vi "Auto.vi"() -> ()   [LabVIEW 2020]
uses:
  Global_Variable/Global.vi
  Global_Variable/A180648.vi
  Global_Variable/System_Conf.vi
  Libraries/S7/S7.lvlib
panel:
  out "前序":string
  out "用户事件输出":refnum<user-event>
  out "磨合正向初始化":bool
  out "工位三开始计时1":bool
  out "产品变更_Event":refnum<user-event>
  out "T1+T2":dbl
  out "T2":dbl
  out "T1":dbl
  out "吸收电流":sgl
  out "输出扭矩(大)":sgl
  out "输入扭矩":sgl
  out "力特性逆向去程":bool
  out "力特性正向去程":bool
  out "力特性逆向回程":bool
  out "力特性正向回程":bool
  out "工位三开始计时":bool
  out "工位二开始计时":bool
  out "功能正向初始化":bool
  out "功能逆向初始化":bool
  out "空载逆向初始化":bool
  out "空载正向初始化":bool
  out "试验项目":T1(tab)
  out "拉压曲线":cluster{dbl[], dbl[]}[](graph)
  out "侧铆曲线":cluster{dbl[], dbl[]}[](graph)
  out "0°曲线":cluster{dbl[], dbl[]}[](graph)
  out "45°曲线":cluster{dbl[], dbl[]}[](graph)
  out "力特性试验":cluster{dbl[], dbl[]}[](graph)
  out "功能试验":cluster{dbl[], dbl[]}[](graph)
  out "电流特性试验":cluster{dbl[], dbl[]}[](graph)
  out "逆向空载试验":cluster{dbl[], dbl[]}[](graph)
  out "磨合":cluster{dbl[], dbl[]}[](graph)
  in  "判定结果":bool[][](array[boolean])=[[TRUE]]
  in  "STEP":string
  # "车速0"
  # "车速1"
  # "车速2"
  # "车速3"
  # "车速4"
  # "车速5"
  # "车速0"
  # "车速1"
  # "车速2"
  # "车速3"
  # "车速4"
  # "车速5"
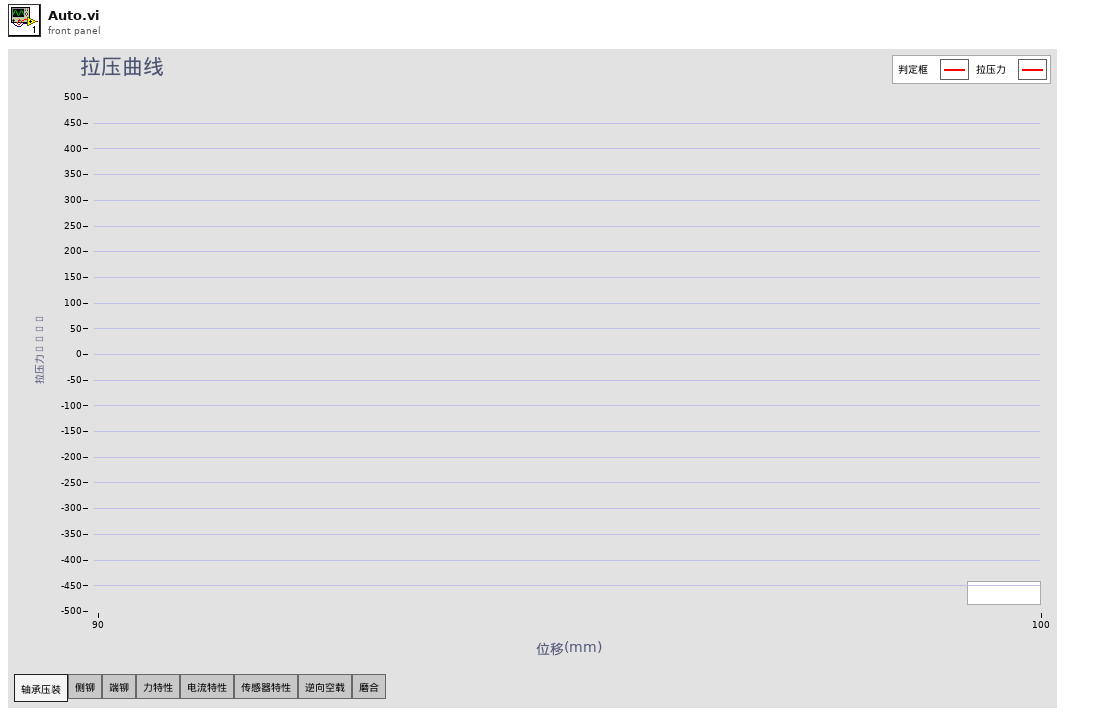
[diagram p1: front panel]
types:
  T1 = enum32{"轴承压装", "侧铆", "端铆", "力特性", "电流特性", "传感器特性", "逆向空载", "磨合"}
  T2 = enum32{"Invalid", "Standard", "Closed", "Hidden", "Minimized", "Maximized"}
  T3 = cluster{"输入轴扭矩":dbl, "输出轴扭矩小量程":dbl, "输出轴扭矩大量程":dbl}
  T4 = typedef "System_conf.ctl" = cluster{"空载滤波":bool, "逆向空载滤波":bool, "空载扭矩系数":dbl, "逆向空载扭矩系数":dbl}
  T5 = cluster{"位移":cluster{"单位":string, "下限":dbl, "上限":dbl}, "压力":cluster{"单位":string, "下限":dbl, "上限":dbl}}
  T6 = cluster{"压最大值":cluster{"单位":string, "下限":dbl, "上限":dbl}, "压力最小值":cluster{"单位":string, "下限":dbl, "上限":dbl}, "拉力最大值":cluster{"单位":string, "下限":dbl, "上限":dbl}, "拉力最小值":cluster{"单位":string, "下限":dbl, "上限":dbl}}
  T7 = cluster{"输入旋转位移":sgl, "电缸位移":sgl, "工装移载位移":sgl, "电缸位移":sgl, "输入扭矩":sgl, "拉压力":sgl, "输出扭矩(大)":sgl, "电缸压力":sgl}
  T8 = typedef "lveventtype.ctl" = enum32{"Null", "Timeout", "Annotation Menu Selection", "Annotation Menu Selection?", "App Instance Close", "App Instance Close?", "Autoscale Range Change", "Bookmark Info Change", "Cell Edit", "Cell Edit?", "Cursor Grab", "Cursor Grab?", "Cursor Menu Selection", "Cursor Menu Selection?", "Cursor Move", "Cursor Release", "Data Change", "Direction Change", "Display State Change", "Drag Ended", "Drag Enter", "Drag Leave", "Drag Over", "Drag Source Update", "Drag Starting", "Drag Starting?", "Drop", "Exec State Change", "Key Down", "Key Down?", "Key Repeat", "Key Repeat?", "Key Up", "Listbox Double Click", "Menu Activation?", "Menu Selection (App)", "Menu Selection? (App)", "Menu Selection (User)", "Mouse Down", "Mouse Down?", "Mouse Enter", "Mouse Leave", "Mouse Move", "Mouse Up", "Mouse Wheel", "NI Security User Change (App)", "Pane Size", "Panel Close", "Panel Close?", "Panel Resize", "Plot Attribute Change", "Scale Range Change", "Shortcut Menu Activation?", "Shortcut Menu Selection (App)", "Shortcut Menu Selection? (App)", "Shortcut Menu Selection (User)", "Tree Double Click", "Tree Drag", "Tree Drag?", "Tree Drop", "Tree Drop?", "Tree Item Close", "Tree Item Close?", "Tree Item Open", "Tree Item Open?", "User Event", "Value Change"}
  T9 = typedef "LVPoint32TypeDef.ctl" = cluster{"Horizontal":i32, "Vertical":i32}
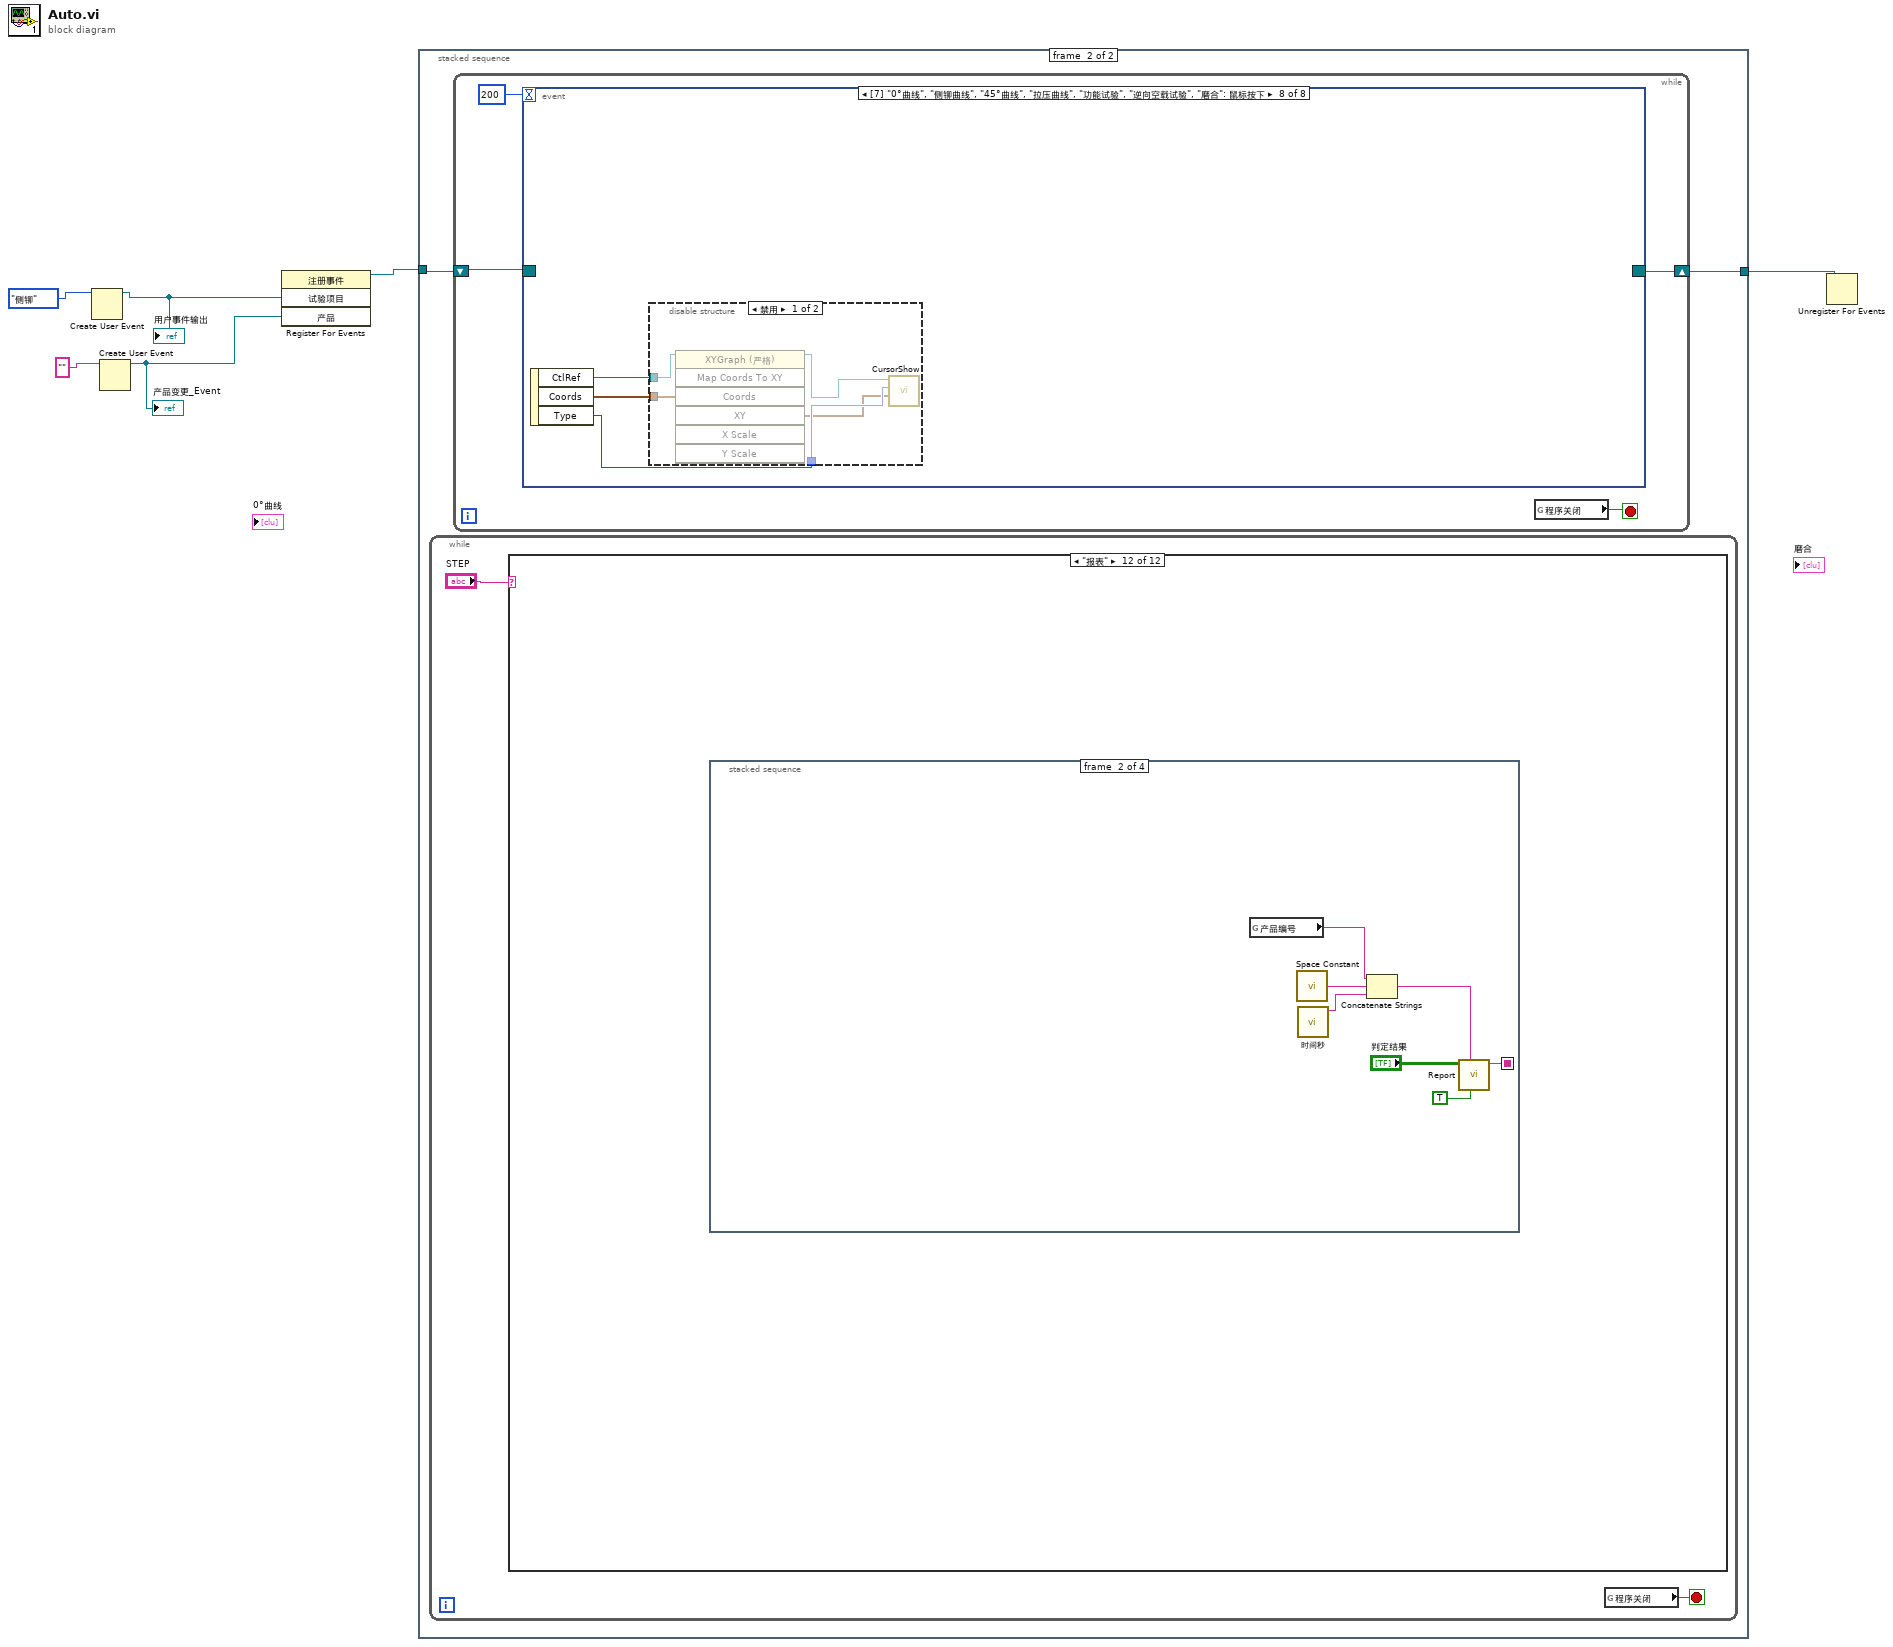
[diagram p0: block diagram]
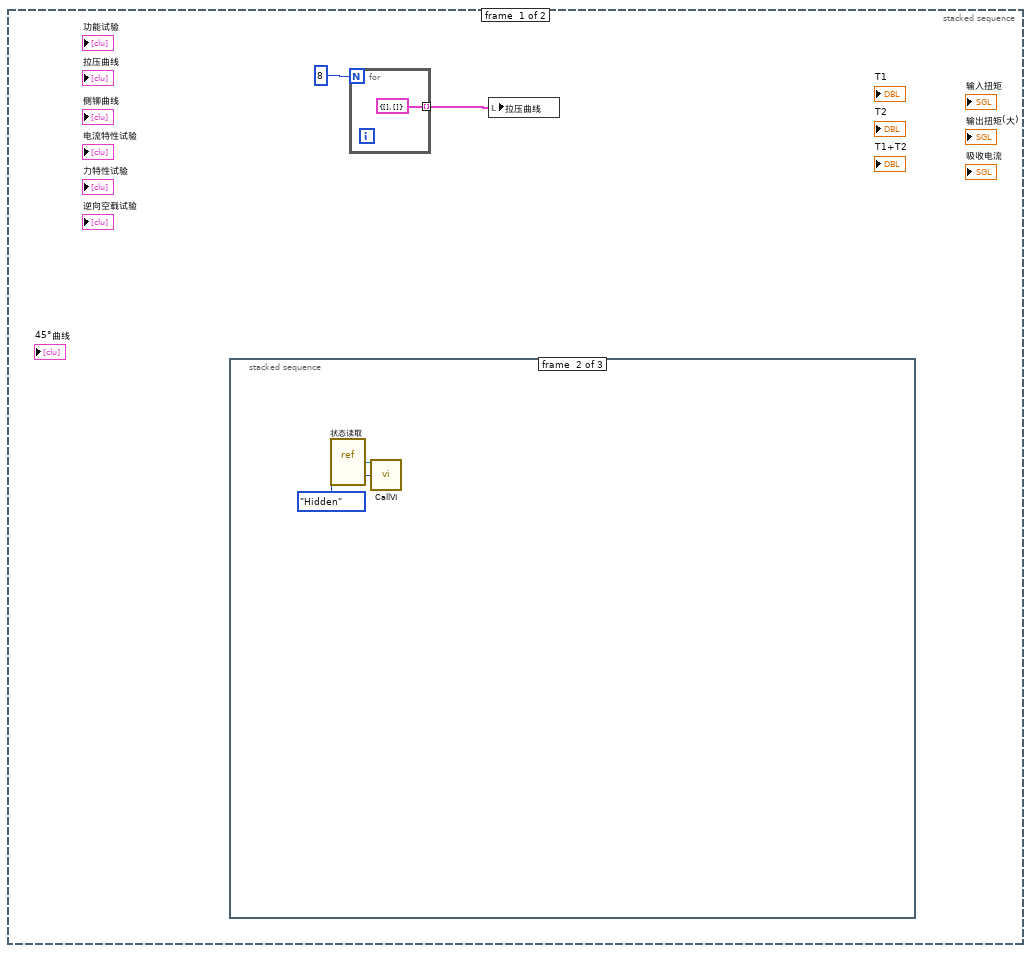
[diagram p2: hidden frame]
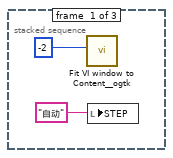
[diagram p3: hidden frame]
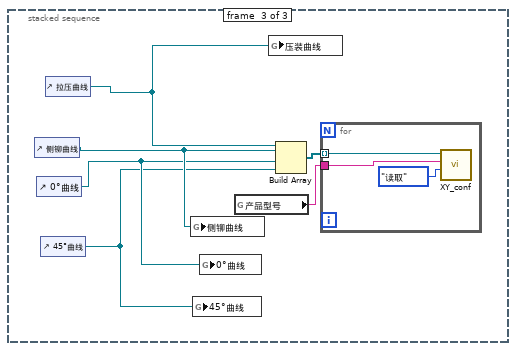
[diagram p4: hidden frame]
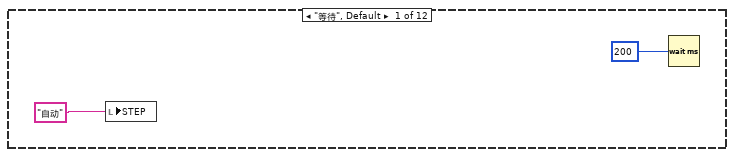
[diagram p5: hidden frame]
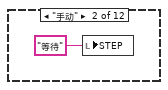
[diagram p6: hidden frame]
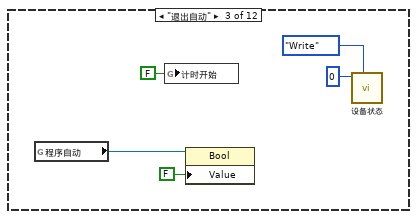
[diagram p7: hidden frame]
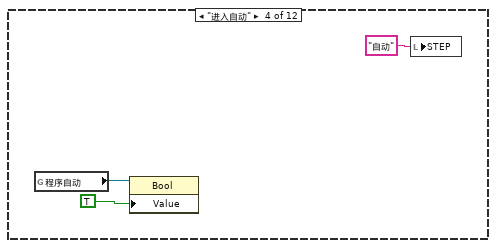
[diagram p8: hidden frame]
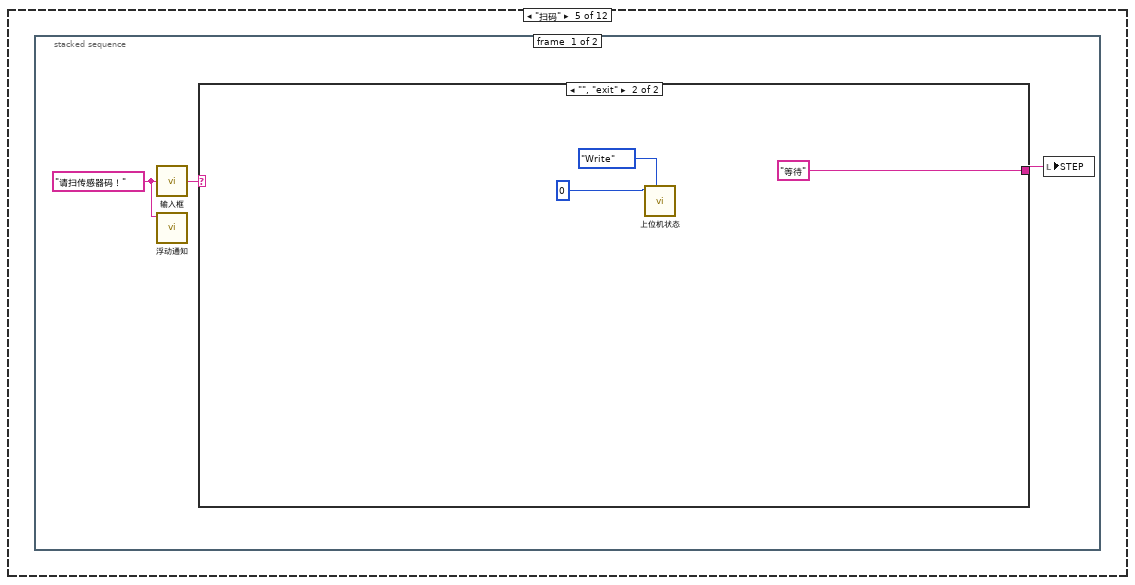
[diagram p9: hidden frame]
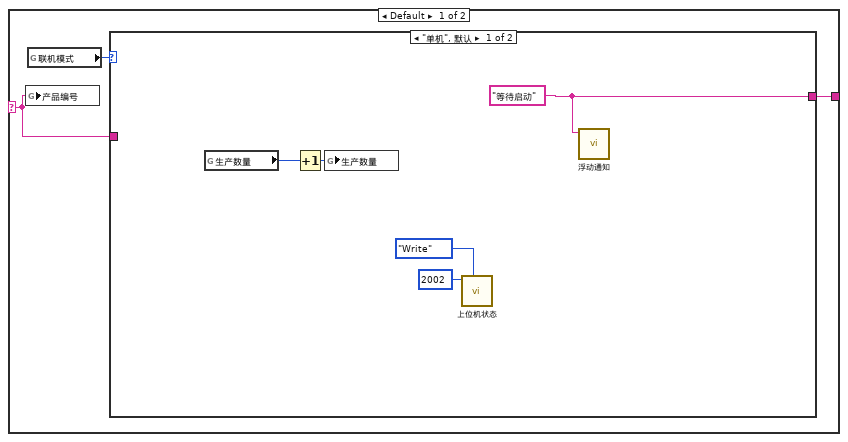
[diagram p10: hidden frame]
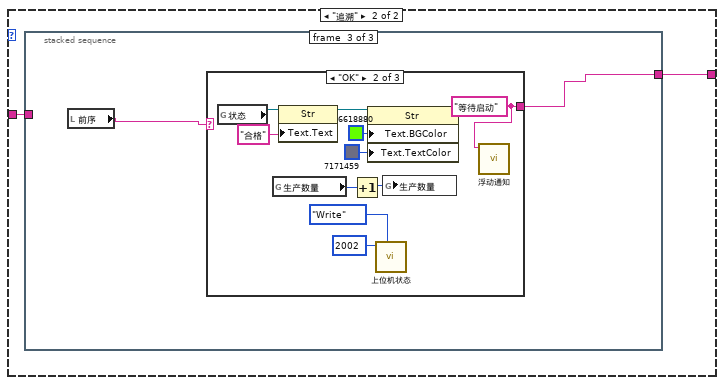
[diagram p11: hidden frame]
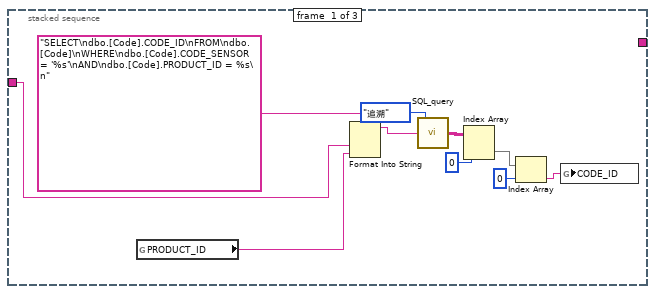
[diagram p12: hidden frame]
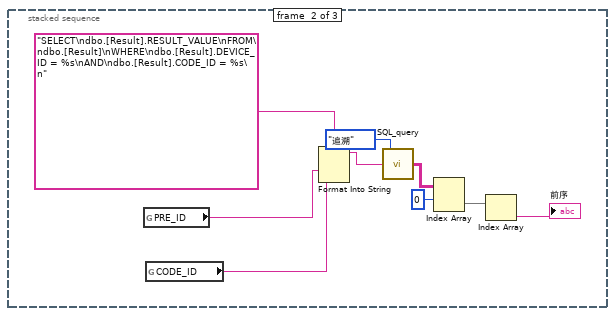
[diagram p13: hidden frame]
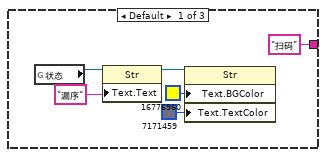
[diagram p14: hidden frame]
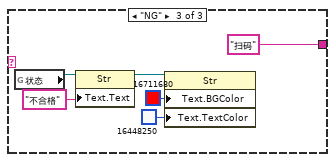
[diagram p15: hidden frame]
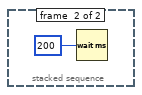
[diagram p16: hidden frame]
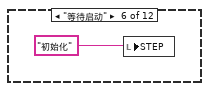
[diagram p17: hidden frame]
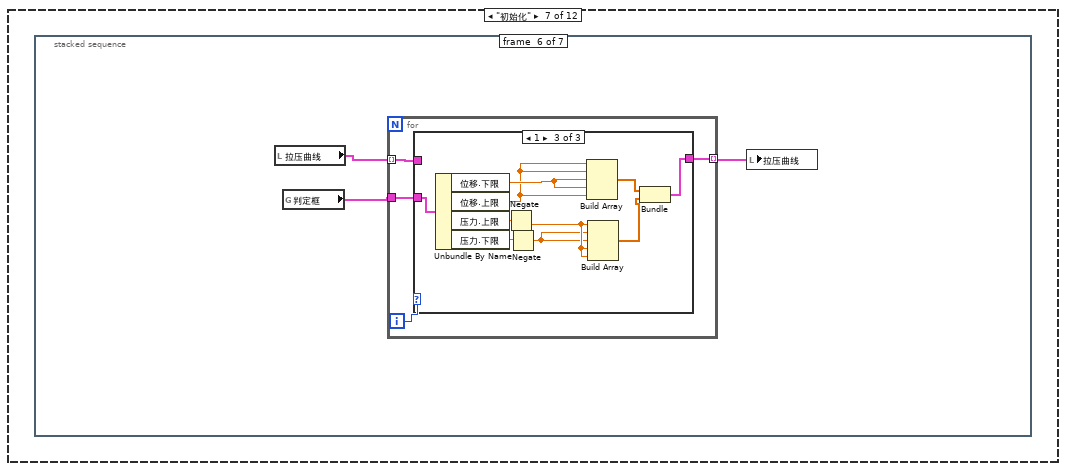
[diagram p18: hidden frame]
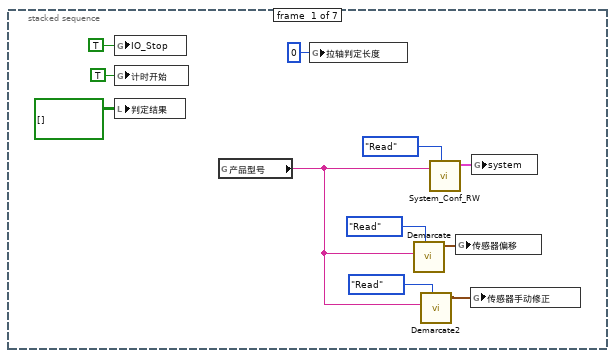
[diagram p19: hidden frame]
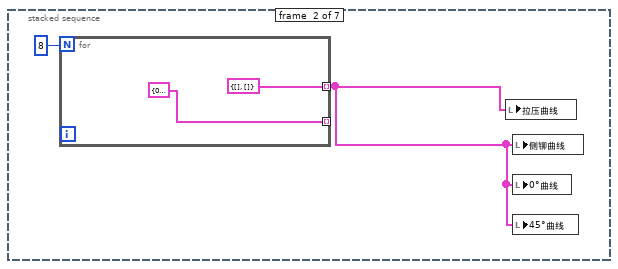
[diagram p20: hidden frame]
diagram:
  n1 = Create User Event(user event datatype=T1."侧铆" ("试验项目")) -> (user event=w1:refnum<user-event>)  [unwired: 1 in, 1 out]
  "用户事件输出" <- w1
  n2 = Create User Event(user event datatype="" ("产品")) -> (user event=w3:refnum<user-event>)  [unwired: 1 in, 1 out]
  "产品变更_Event" <- w3
  n3 = register-events(w1, w3) -> (reference out=w6:refnum<event-registration>)  [unwired: 2 in, 1 out]
  n4 = stacked-sequence {
    tunnel: w6 -> [_ w24]
    tunnel: [_ w23] -> w5
    frame #0 {
      n5 = stacked-sequence {
        frame #0 {
          n6 = call <userlib>:"Fit VI window to Content__ogtk.vi"("border spacing (2 px)"=-2) -> ()  [unwired: 5 in, 2 out]
          n7 = local write "STEP"("自动" ("STEP")) -> ()
        }
        frame #1 {
          n8 = vi-ref "状态读取.vi"() -> (w13:refnum<vi>)
          n9 = call "CallVI.vi"("VI引用"=w13, "状态"=T2."Hidden") -> ()  [unwired: 12 in, 2 out]
        }
        frame #2 {
          n10 = control-ref of="侧铆曲线"() -> (w17:refnum<vi>)
          n11 = control-ref of="0°曲线"() -> (w16:refnum<vi>)
          n12 = control-ref of="45°曲线"() -> (w15:refnum<vi>)
          n13 = control-ref of="拉压曲线"() -> (w14:refnum<vi>)
          n14 = global write "A180648.vi" "侧铆曲线"(w17) -> ()
          n15 = global write "A180648.vi" "45°曲线"(w15) -> ()
          n16 = global write "A180648.vi" "0°曲线"(w16) -> ()
          n17 = global read "Global.vi" "产品型号"() -> (w18:string)
          n18 = global write "A180648.vi" "压装曲线"(w14) -> ()
          n19 = Build Array(w14, w17, w16, w15) -> (w19:refnum<vi>[])
          n20 = for {
            tunnel: w19 -> [w21] mode=indexing
            tunnel: w18 -> [w20]
            n21 = call "XY_conf.vi"("方式"=enum16{"写入", "读取"}."读取", "产品"=w20, "XY图引用"=w21) -> ()  [unwired: 4 in, 1 out]
          }
        }
      }
      n22 = for {
        N: 8 -> [_]
        tunnel: [cluster{dbl[], dbl[]} {[], []}] -> w8 mode=indexing
      }
      n23 = local write "拉压曲线"(w8) -> ()
    }
    frame #1 {
      n24 = while {
        stop <- w26 stop-if-true
        n25 = case shown="\"报表\"" "STEP" {
          frame "等待", Default {
            n26 = local write "STEP"("自动" ("STEP")) -> ()
            n27 = Wait (ms)(milliseconds to wait=u32 200 ("等待时间（毫秒）")) -> ()  [unwired: 1 out]
          }
          frame "手动" {
            n28 = local write "STEP"("等待" ("STEP")) -> ()
          }
          frame "退出自动" {
            n29 = global read "Global.vi" "程序自动"() -> (w31:refnum<vi>)
            n30 = global write "Global.vi" "计时开始"(FALSE ("计时开始")) -> ()
            n31 = property class="Bool"(reference=w31, "Value"=FALSE) -> ()  [unwired: 1 in, 2 out]
            n32 = call "设备状态.vi"("枚举"=enum16{"Read", "Write"}."Write", "Status_Write"=i16 0) -> ()  [unwired: 9 in, 1 out]
          }
          frame "进入自动" {
            n33 = global read "Global.vi" "程序自动"() -> (w36:refnum<vi>)
            n34 = property class="Bool"(reference=w36, "Value"=TRUE) -> ()  [unwired: 1 in, 2 out]
            n35 = local write "STEP"("自动" ("STEP")) -> ()
          }
          frame "扫码" {
            n36 = stacked-sequence {
              frame #0 {
                w39 = "请扫传感器码！" ("提示信息")
                n37 = call "输入框.vi"("提示信息"=w39) -> ("条形码输出"=w40:string)
                n38 = call "浮动通知.vi"("通知内容"=w39) -> ()  [unwired: 11 in]
                n39 = case shown="\"\", \"exit\"" w40 {
                  selector: w40 -> [w41 _]
                  tunnel: [w43 "等待" ("State(s) in Front (\"\")")] -> w38
                  frame Default {
                    n40 = global write "Global.vi" "产品编号"(w41) -> ()
                    n41 = global read "Global.vi" "联机模式"() -> (w42:enum16{"单机", "追溯"})
                    n42 = case shown="\"单机\", 默认" w42 {
                      tunnel: [w46 w50] -> w43
                      tunnel: w41 -> [_ w49]
                      frame "单机", Default {
                        w46 = "等待启动" ("State(s) in Front (\"\")")
                        n43 = global read "Global.vi" "生产数量"() -> (w47:i32)
                        n44 = Increment(x=w47) -> (x+1=w48:i32)
                        n45 = global write "Global.vi" "生产数量"(w48) -> ()
                        n46 = call "上位机状态.vi"("枚举"=enum16{"Read", "Write"}."Write", "Status_Write"=i16 2002) -> ()  [unwired: 9 in, 1 out]
                        n47 = call "浮动通知.vi"("通知内容"=w46) -> ()  [unwired: 11 in]
                      }
                      frame "追溯" {
                        n48 = stacked-sequence {
                          tunnel: [_ _ w71] -> w50
                          tunnel: w49 -> [w59 _ _]
                          frame #0 {
                            n49 = global read "追溯Global.vi" "PRODUCT_ID"() -> (w58:string)
                            n50 = Format Into String(format string="SELECT\ndbo.[Code].CODE_ID\nFROM\ndbo.[Code]\nWHERE\ndbo.[Code].CODE_SENSOR = '%s'\nAND\ndbo.[Code].PRODUCT_ID = %s\n" ("格式字符串"), w59, w58) -> (resulting string=w57:string)  [unwired: 2 in, 1 out]
                            n51 = call "SQL_query.vi"("SQL query"=w57, "联机模式"=enum16{"单机", "追溯"}."追溯") -> ("data"=w55:string[][])  [unwired: 2 in, 1 out]
                            n52 = Index Array(array=w55, index (row)=0 ("索引 (行)")) -> (element=w53:string[])  [unwired: 1 in]
                            n53 = Index Array(array=w53, index=0 ("索引")) -> (element=w51:string)
                            n54 = global write "追溯Global.vi" "CODE_ID"(w51) -> ()
                          }
                          frame #1 {
                            n55 = global read "追溯Global.vi" "PRE_ID"() -> (w68:string)
                            n56 = global read "追溯Global.vi" "CODE_ID"() -> (w67:string)
                            n57 = Format Into String(format string="SELECT\ndbo.[Result].RESULT_VALUE\nFROM\ndbo.[Result]\nWHERE\ndbo.[Result].DEVICE_ID = %s\nAND\ndbo.[Result].CODE_ID = %s\n" ("格式字符串"), w68, w67) -> (resulting string=w66:string)  [unwired: 2 in, 1 out]
                            n58 = call "SQL_query.vi"("SQL query"=w66, "联机模式"=enum16{"单机", "追溯"}."追溯") -> ("data"=w64:string[][])  [unwired: 2 in, 1 out]
                            n59 = Index Array(array=w64, index (row)=0 ("索引 (行)")) -> (element=w62:string[])  [unwired: 1 in]
                            n60 = Index Array(array=w62) -> (element=→"前序":string)  [unwired: 1 in]
                          }
                          frame #2 {
                            n61 = local read "前序"() -> (w70:string)
                            n62 = case shown="\"OK\"" w70 {
                              tunnel: ["扫码" ("State(s) in Front (\"\")") w82 "扫码" ("State(s) in Front (\"\")")] -> w71
                              frame Default {
                                n63 = global read "Global.vi" "状态"() -> (w77:refnum<vi>)
                                n64 = property class="Str"(reference=w77, "Text.Text"="漏序" ("文本.文本")) -> (reference out=w76:refnum<vi>)  [unwired: 1 in, 1 out]
                                n65 = property class="Str"(reference=w76, "Text.BGColor"=u32 16776960 ("文本.文本颜色:背景色"), "Text.TextColor"=u32 7171459 ("文本.文本颜色:文本颜色")) -> ()  [unwired: 1 in, 2 out]
                              }
                              frame "OK" {
                                w82 = "等待启动" ("State(s) in Front (\"\")")
                                n66 = global read "Global.vi" "状态"() -> (w87:refnum<vi>)
                                n67 = global read "Global.vi" "生产数量"() -> (w80:i32)
                                n68 = property class="Str"(reference=w87, "Text.Text"="合格" ("文本.文本")) -> (reference out=w85:refnum<vi>)  [unwired: 1 in, 1 out]
                                n69 = Increment(x=w80) -> (x+1=w81:i32)
                                n70 = property class="Str"(reference=w85, "Text.BGColor"=u32 6618880 ("文本.文本颜色:背景色"), "Text.TextColor"=u32 7171459 ("文本.文本颜色:文本颜色")) -> ()  [unwired: 1 in, 2 out]
                                n71 = call "上位机状态.vi"("枚举"=enum16{"Read", "Write"}."Write", "Status_Write"=i16 2002) -> ()  [unwired: 9 in, 1 out]
                                n72 = global write "Global.vi" "生产数量"(w81) -> ()
                                n73 = call "浮动通知.vi"("通知内容"=w82) -> ()  [unwired: 11 in]
                              }
                              frame "NG" {
                                n74 = global read "Global.vi" "状态"() -> (w93:refnum<vi>)
                                n75 = property class="Str"(reference=w93, "Text.Text"="不合格" ("文本.文本")) -> (reference out=w91:refnum<vi>)  [unwired: 1 in, 1 out]
                                n76 = property class="Str"(reference=w91, "Text.BGColor"=u32 16711680 ("文本.文本颜色:背景色"), "Text.TextColor"=u32 16448250 ("文本.文本颜色:文本颜色")) -> ()  [unwired: 1 in, 2 out]
                              }
                            }
                          }
                        }
                      }
                    }
                  }
                  frame "", "exit" {
                    n77 = call "上位机状态.vi"("枚举"=enum16{"Read", "Write"}."Write", "Status_Write"=u16 0 ("设备状态")) -> ()  [unwired: 9 in, 1 out]
                  }
                }
                n78 = local write "STEP"(w38) -> ()
              }
              frame #1 {
                n79 = Wait (ms)(milliseconds to wait=u32 200 ("等待时间（毫秒）")) -> ()  [unwired: 1 out]
              }
            }
          }
          frame "等待启动" {
            n80 = local write "STEP"("初始化" ("STEP")) -> ()
          }
          frame "初始化" {
            n81 = stacked-sequence {
              frame #0 {
                n82 = global write "Global.vi" "IO_Stop"(TRUE ("IO_Stop")) -> ()
                n83 = global write "Global.vi" "计时开始"(TRUE ("计时开始")) -> ()
                n84 = local write "判定结果"(bool[][] [] ("判定结果")) -> ()
                n85 = global read "Global.vi" "产品型号"() -> (w100:string)
                n86 = global write "判定参数.vi" "拉轴判定长度"(0 ("拉轴判定长度")) -> ()
                n87 = call "Demarcate.vi"("Mode"=enum16{"Read", "Write"}."Read", "Section"=w100) -> ("Sensor OUT"=w104:T3)  [unwired: 8 in, 1 out]
                n88 = call "Demarcate2.vi"("Mode"=enum16{"Read", "Write"}."Read", "Section"=w100) -> ("Sensor OUT"=w103:T3)  [unwired: 8 in, 1 out]
                n89 = call "System_Conf_RW.vi"("Mode"=enum16{"Read", "Write"}."Read", "Section"=w100) -> ("system_out"=w106:T4)  [unwired: 8 in, 1 out]
                n90 = global write "传感器偏移.vi" "传感器偏移"(w104) -> ()
                n91 = global write "传感器偏移.vi" "传感器手动修正"(w103) -> ()
                n92 = global write "System_Conf.vi" "system"(w106) -> ()
              }
              frame #1 {
                n93 = for {
                  N: 8 -> [_]
                  tunnel: [cluster{dbl[], dbl[]} {[], []}] -> w110 mode=indexing
                  tunnel: [cluster{"f0":dbl, "df":dbl, "magnitude":dbl[]} {"f0"=0.0, "df"=0.0, "magnitude"=[]} ("power spectrum [dB EU]")] -> _ mode=indexing
                }
                n94 = local write "拉压曲线"(w110) -> ()
                n95 = local write "侧铆曲线"(w110) -> ()
                n96 = local write "0°曲线"(w110) -> ()
                n97 = local write "45°曲线"(w110) -> ()
              }
              frame #2 {
                w115 = -2
                n98 = global read "Global.vi" "Result"() -> (w117:refnum<vi>)
                n99 = Bundle(w115, w115) -> (w114:cluster{i32, i32})  [unwired: 1 in]
                n100 = property class="Tbl"(reference=w117, "Active Cell"=w114, "Cell BG Color"=u32 16777216 ("活动单元格:单元格背景色")) -> ()  [unwired: 1 in, 2 out]
                n101 = property class="Tbl"(reference=w117, "Value"=string[][] []) -> (reference out=w120:refnum<vi>, error out=w121:errorcluster)  [unwired: 1 in]
                n102 = property class="Tbl"(reference=w120, error in=w121, "Row Headers[]"=string[] [] ("列首字符串[]")) -> ()  [unwired: 2 out]
              }
              frame #3 {
                n103 = global read "A180648.vi" "LED-轴承压装"() -> (w125:refnum<vi>)
                n104 = global read "A180648.vi" "LED-端铆"() -> (w122:refnum<vi>)
                n105 = global read "A180648.vi" "LED-侧铆"() -> (w123:refnum<vi>)
                n106 = Build Array(w125, w123, w122) -> (w124:refnum<vi>[])
                n107 = for {
                  tunnel: w124 -> [w126] mode=indexing
                  n108 = property class="Bool"(reference=w126, "Colors [4]"=cluster{u32, u32}[] [{12369084, 12369084}] ("颜色[4]")) -> ()  [unwired: 1 in, 2 out]
                }
              }
              frame #4 {
                w129 = 1 ("维数大小")
                n109 = Initialize Array(" " ("字符串"), w129, w129, w129) -> (w131:string[][][])
                n110 = global write "A180648.vi" "当前检测项"(enum32{"拉轴", "卡簧", "完成"}."拉轴" ("当前检测项")) -> ()
                n111 = global write "A180648.vi" "检测结果"(w131) -> ()
              }
              frame #5 {
                n112 = local read "拉压曲线"() -> (w133:cluster{dbl[], dbl[]}[])
                n113 = global read "判定参数.vi" "判定框"() -> (w134:T5)
                n114 = for {
                  tunnel: w133 -> [w137] mode=indexing
                  tunnel: [w136] -> w132 mode=indexing
                  tunnel: w134 -> [w135]
                  i -> [w138]
                  n115 = case shown="1" w138 {
                    tunnel: w137 -> [w139 _ _]
                    tunnel: [w139 w142 w152] -> w136
                    tunnel: w135 -> [_ w147 w157]
                    frame Default {
                    }
                    frame 0 {
                      n116 = Unbundle By Name(w147) -> ("位移.下限"=w146:dbl, "位移.上限"=w145:dbl, "压力.下限"=w140:dbl, "压力.上限"=w141:dbl)
                      n117 = Build Array(w145, w145, w146, w146, w145) -> (w144:dbl[])
                      n118 = Build Array(w140, w141, w141, w140, w140) -> (w143:dbl[])
                      n119 = Bundle(w144, w143) -> (w142:cluster{dbl[], dbl[]})  [unwired: 1 in]
                    }
                    frame 1 {
                      n120 = Unbundle By Name(w157) -> ("位移.下限"=w156:dbl, "位移.上限"=w155:dbl, "压力.上限"=w150:dbl, "压力.下限"=w151:dbl)
                      n121 = Negate(x=w150) -> (-x=w149:dbl)
                      n122 = Negate(x=w151) -> (-x=w148:dbl)
                      n123 = Build Array(w155, w155, w156, w156, w155) -> (w154:dbl[])
                      n124 = Build Array(w149, w148, w148, w149, w149) -> (w153:dbl[])
                      n125 = Bundle(w154, w153) -> (w152:cluster{dbl[], dbl[]})  [unwired: 1 in]
                    }
                  }
                }
                n126 = local write "拉压曲线"(w132) -> ()
              }
              frame #6 {
                w159 = TRUE
                n127 = local write "STEP"("自动" ("STEP")) -> ()
                "工位三开始计时" <- w159
                "工位二开始计时" <- w159
                "空载正向初始化" <- w159
                "空载逆向初始化" <- w159
                "功能正向初始化" <- w159
                "功能逆向初始化" <- w159
                "力特性逆向去程" <- w159
                "力特性正向去程" <- w159
                "力特性逆向回程" <- w159
                "力特性正向回程" <- w159
                "磨合正向初始化" <- w159
                "工位三开始计时1" <- w159
              }
            }
          }
          frame "试验项" {
            n128 = global read "A180648.vi" "当前检测项"() -> (w160:enum32{"拉轴", "卡簧", "完成"})
            n129 = case shown="\"拉轴\", 默认" w160 {
              selector: w160 -> [w162 _]
              tunnel: [w165 "报表" ("STEP")] -> w161
              frame "拉轴", Default {
                n130 = global read "Global.vi" "试验项目"() -> (w163:bool[])
                n131 = Index Array(array=w163, index=w162) -> (element=w164:bool)
                n132 = case shown="真" w164 {
                  tunnel: ["试验项" ("字符串") w172] -> w165
                  tunnel: w162 -> [_ w173]
                  frame False {
                    n133 = global read "A180648.vi" "当前检测项"() -> (w170:enum32{"拉轴", "卡簧", "完成"})
                    n134 = Increment(x=w170) -> (x+1=w169:enum32{"拉轴", "卡簧", "完成"})
                    n135 = global write "A180648.vi" "当前检测项"(w169) -> ()
                    n136 = local read "判定结果"() -> (w166:bool[][])
                    n137 = Build Array (concatenate)(w166, bool[] [FALSE] ("判定结果")) -> (w167:bool[][])
                    n138 = local write "判定结果"(w167) -> ()
                  }
                  frame True {
                    n139 = case shown="\"拉轴\", 默认" w173 {
                      tunnel: ["等待" ("STEP") "等待" ("STEP") "报表" ("STEP")] -> w172
                      frame "拉轴", Default {
                        n140 = call "浮动通知.vi"("通知内容"="拉拔力试验") -> ()  [unwired: 11 in]
                        n141 = property on="试验项目" class="TabCtl (严格)"("Val(Sgnl)"=T1."轴承压装" ("值(信号)")) -> ()  [unwired: 2 in, 2 out]
                      }
                      frame "卡簧" {
                        n142 = call "浮动通知.vi"("通知内容"="卡簧检测") -> ()  [unwired: 11 in]
                      }
                      frame "完成" {
                      }
                    }
                  }
                }
              }
              frame "完成" {
              }
            }
            n143 = local write "STEP"(w161) -> ()
          }
          frame "判定" {
            n144 = stacked-sequence {
              frame #0 {
                n145 = global read "判定参数.vi" "拉压判定参数"() -> (w192:T6)
                n146 = local read "拉压曲线"() -> (w193:cluster{dbl[], dbl[]}[])
                n147 = global read "Global.vi" "Result"() -> (w191:refnum<vi>)
                n148 = call "压装试验判定.vi"("Result"=w191, "判定参数"=w192, "XY曲线"=w193) -> ("判定项长度"=w182:i32, "OK？"=w181:bool)  [unwired: 7 in]
                n149 = global read "A180648.vi" "LED-轴承压装"() -> (w187:refnum<vi>)
                n150 = local read "判定结果"() -> (w183:bool[][])
                n151 = Select(t=cluster{u32, u32}[] [{6618880, 6618880}, {6618880, 6618880}, {6618880, 6618880}, {6618880, 6618880}] ("颜色[4]"), s=w181, f=cluster{u32, u32}[] [{16711680, 16711680}, {16711680, 16711680}, {16711680, 16711680}, {16711680, 16711680}] ("颜色[4]")) -> (s? t:f=w188:cluster{u32, u32}[])
                n152 = Build Array(TRUE, w181) -> (w186:bool[])
                n153 = global write "判定参数.vi" "拉轴判定长度"(w182) -> ()
                n154 = property class="Bool"(reference=w187, "Colors [4]"=w188) -> ()  [unwired: 1 in, 2 out]
                n155 = Build Array (concatenate)(w183, w186) -> (w184:bool[][])
                n156 = case shown="真" w181 {
                  frame False {
                    n157 = shared-variable "我的电脑\\Modbus_Rapid.lvlib\\工位1合格状态"(u16 2 ("工位1合格状态")) -> ()  [unwired: 1 in, 1 out]
                  }
                  frame True {
                    n158 = shared-variable "我的电脑\\Modbus_Rapid.lvlib\\工位1合格状态"(u16 1 ("工位1合格状态")) -> ()  [unwired: 1 in, 1 out]
                  }
                }
                n159 = local write "判定结果"(w184) -> ()
              }
              frame #1 {
                n160 = local write "STEP"("报表") -> ()
              }
            }
          }
          frame "自动" {
            n161 = global read "Global.vi" "设备状态"() -> (w199:i16)
            n162 = case shown="1024" w199 {
              frame -128 {
                n163 = global write "Global.vi" "计时开始"(FALSE ("计时开始")) -> ()
                n164 = call "浮动通知.vi"("通知内容"="复位中……" ("Status")) -> ()  [unwired: 11 in]
              }
              frame Default {
              }
              frame 0 {
                n165 = disable-structure shown="禁用" {
                  frame Disabled {
                    n166 = global write "Global.vi" "计时开始"(FALSE ("计时开始")) -> ()
                  }
                  frame Enabled {
                  }
                }
              }
              frame 1 {
                n167 = disable-structure shown="禁用" {
                  frame Disabled {
                    n168 = local read "拉压曲线"() -> (w241:cluster{dbl[], dbl[]}[])
                    n169 = for {
                      tunnel: [w243] -> _ mode=indexing
                      tunnel: w241 -> [w242] mode=indexing
                      i -> [w244]
                      n170 = case shown="2" w244 {
                        tunnel: [_ w245] -> w243
                        tunnel: w242 -> [_ w250]
                        frame Default {
                        }
                        frame 2 {
                          n171 = Unbundle(w250) -> (w249:dbl[], w248:dbl[])
                          n172 = Build Array(w249) -> (w247:dbl[][])  [unwired: 1 in]
                          n173 = Build Array(w248) -> (w246:dbl[][])  [unwired: 1 in]
                          n174 = Bundle(w247, w246) -> (w245:cluster{dbl[][], dbl[][]})  [unwired: 1 in]
                        }
                      }
                    }
                    n175 = local read "拉压曲线"() -> ()  [unwired: 1 in]
                  }
                  frame Enabled {
                  }
                }
              }
              frame 2 {
              }
              frame 5 {
                n176 = call "浮动通知.vi"("通知内容"="复位完成" ("Status")) -> ()  [unwired: 11 in]
              }
              frame 8 {
                n177 = call "浮动通知.vi"("通知内容"="程序停止！" ("Status")) -> ()  [unwired: 11 in]
              }
              frame 100 {
                n178 = call "浮动通知.vi"("通知内容"="压紧气缸伸出！" ("Status")) -> ()  [unwired: 11 in]
              }
              frame 20 {
              }
              frame 105 {
                n179 = call "浮动通知.vi"("通知内容"="压紧缸下降！" ("Status")) -> ()  [unwired: 11 in]
              }
              frame 120 {
                n180 = call "浮动通知.vi"("通知内容"="夹爪夹紧！" ("Status")) -> ()  [unwired: 11 in]
              }
              frame 130 {
                n181 = call "浮动通知.vi"("通知内容"="拉升磨合" ("Status")) -> ()  [unwired: 11 in]
              }
              frame 161 {
                n182 = call "浮动通知.vi"("通知内容"="夹爪松开" ("Status")) -> ()  [unwired: 11 in]
                n183 = local write "STEP"("判定" ("STEP")) -> ()
              }
              frame 163 {
                n184 = call "浮动通知.vi"("通知内容"="请取记号笔" ("Status")) -> ()  [unwired: 11 in]
              }
              frame 10 {
              }
              frame 999 {
                n185 = call "浮动通知.vi"("通知内容"="请启动！" ("Status")) -> ()  [unwired: 11 in]
              }
              frame 1000 {
              }
              frame 1002 {
              }
              frame 1024 {
                n186 = local write "STEP"("退出自动" ("STEP")) -> ()
              }
            }
            n187 = call "上位机状态.vi"("枚举"=enum16{"Read", "Write"}."Read") -> ("Status_Read"=w198:i16)  [unwired: 10 in]
            n188 = case shown="5" w198 {
              frame 0, Default {
              }
              frame 2000 {
                n189 = local write "STEP"("扫码" ("STEP")) -> ()
              }
              frame 4 {
                n190 = local write "STEP"("初始化" ("STEP")) -> ()
              }
              frame 5 {
                n191 = local read "拉压曲线"() -> (w202:cluster{dbl[], dbl[]}[])
                n192 = global read "判定参数.vi" "判定框"() -> (w204:T5)
                n193 = for {
                  tunnel: w202 -> [w207] mode=indexing
                  tunnel: [w206] -> w203 mode=indexing
                  tunnel: w204 -> [w205]
                  i -> [w208]
                  n194 = case shown="1" w208 {
                    tunnel: w207 -> [w209 _ _]
                    tunnel: [w209 w212 w222] -> w206
                    tunnel: w205 -> [_ w217 w223]
                    frame Default {
                    }
                    frame 0 {
                      n195 = Unbundle By Name(w217) -> ("位移.下限"=w216:dbl, "位移.上限"=w215:dbl, "压力.下限"=w210:dbl, "压力.上限"=w211:dbl)
                      n196 = Build Array(w215, w215, w216, w216, w215) -> (w214:dbl[])
                      n197 = Build Array(w210, w211, w211, w210, w210) -> (w213:dbl[])
                      n198 = Bundle(w214, w213) -> (w212:cluster{dbl[], dbl[]})  [unwired: 1 in]
                    }
                    frame 1 {
                      n199 = Unbundle By Name(w223) -> ("位移.下限"=w227:dbl, "位移.上限"=w226:dbl, "压力.上限"=w220:dbl, "压力.下限"=w221:dbl)
                      n200 = Negate(x=w221) -> (-x=w218:dbl)
                      n201 = Negate(x=w220) -> (-x=w219:dbl)
                      n202 = Build Array(w226, w226, w227, w227, w226) -> (w225:dbl[])
                      n203 = Build Array(w219, w218, w218, w219, w219) -> (w224:dbl[])
                      n204 = Bundle(w225, w224) -> (w222:cluster{dbl[], dbl[]})  [unwired: 1 in]
                    }
                  }
                }
                n205 = local write "拉压曲线"(w203) -> ()
              }
              frame 1 {
                n206 = global read "Global.vi" "传感器读数"() -> (w230:T7)
                n207 = Unbundle By Name(w230) -> ("电缸位移"=w229:sgl, "拉压力"=w228:sgl)
                n208 = control-ref of="拉压曲线"() -> (w232:refnum<vi>)
                n209 = call "曲线采集.vi"("曲线引用"=w232, "曲线索引"=2, "X"=w229, "Y"=w228) -> ()  [unwired: 10 in, 2 out]
              }
              frame 2 {
                n210 = global read "Global.vi" "传感器读数"() -> (w235:T7)
                n211 = Unbundle By Name(w235) -> ("电缸位移"=w234:sgl, "拉压力"=w233:sgl)
                n212 = control-ref of="拉压曲线"() -> (w237:refnum<vi>)
                n213 = call "曲线采集.vi"("曲线引用"=w237, "曲线索引"=3, "X"=w234, "Y"=w233) -> ()  [unwired: 10 in, 2 out]
              }
            }
          }
          frame "合格判定" {
            n214 = Wait (ms)(milliseconds to wait=u32 100 ("等待时间（毫秒）")) -> ()  [unwired: 1 out]
            n215 = local write "STEP"("等待" ("STEP")) -> ()
          }
          frame "报表" {
            n216 = stacked-sequence {
              seq-local: [_ w271 _ _] -> [_ _ w275 _]
              frame #0 {
                n217 = global write "Global.vi" "计时开始"(FALSE ("计时开始")) -> ()
                n218 = disable-structure shown="禁用" {
                  frame Disabled {
                    n219 = global read "Global.vi" "产品编号"() -> (w266:string)
                    n220 = call "Get_CODE_ID.vi"("CODE_MAIN"=w266) -> ("CODE_ID"=w265:string)  [unwired: 10 in]
                    n221 = global write "追溯Global.vi" "CODE_ID"(w265) -> ()
                  }
                  frame Enabled {
                  }
                }
              }
              frame #1 {
                n222 = global read "Global.vi" "产品编号"() -> (w270:string)
                n223 = call <vilib>:"Space Constant.vi"() -> ("String"=w269:string)
                n224 = call "时间秒.vi"() -> ("结果字符串"=w268:string)  [unwired: 11 in]
                n225 = Concatenate Strings(w270, w269, w268) -> (w267:string)
                n226 = call "Report.vi"("文件重命名"=TRUE, "文件名称"=w267, "检测结果"="判定结果") -> ("PRODUCT_VAULE"=w271:string)  [unwired: 7 in, 1 out]
              }
              frame #2 {
                n227 = global read "Global.vi" "联机模式"() -> (w274:enum16{"单机", "追溯"})
                n228 = case shown="\"追溯\"" w274 {
                  tunnel: w275 -> [_ w276]
                  frame "单机", Default {
                  }
                  frame "追溯" {
                    n229 = global read "Global.vi" "Result"() -> (w278:refnum<vi>)
                    n230 = property class="Tbl"(reference=w278) -> (reference out=w283:refnum<vi>, error out=w280:errorcluster, "Row Headers[]"=w281:string[])  [unwired: 1 in]
                    n231 = property class="Tbl"(reference=w283, error in=w280) -> (error out=w279:errorcluster, "Value"=w282:string[][])  [unwired: 1 out]
                    n232 = for {
                      tunnel: w282 -> [w290] mode=indexing
                      tunnel: w281 -> [w291] mode=indexing
                      tunnel: [w288] -> w277 mode=indexing if=w289
                      shift-right: [w287] -> _
                      shift-left: w279 -> [w287]
                      n233 = Build Array (concatenate)(w291, w290) -> (w288:string[])
                      n234 = Index Array(array=w290) -> (element=w292:string)  [unwired: 1 in]
                      n235 = case shown="\"\"" w292 {
                        tunnel: [TRUE FALSE] -> w289
                        frame Default {
                        }
                        frame "" {
                        }
                      }
                    }
                    n236 = global read "追溯Global.vi" "DEVICE_ID"() -> (w285:string)
                    n237 = global read "追溯Global.vi" "CODE_ID"() -> (w286:string)
                    n238 = global read "追溯Global.vi" "USER_ID"() -> (w284:string)
                    n239 = call "UPTEST.vi"("Result"=w277, "CODE_ID"=w286, "DEVICE_ID"=w285) -> ()  [unwired: 6 in, 1 out]
                    n240 = call "UPRESULT.vi"("DEVICE_ID"=w285, "USER_ID"=w284, "CODE_ID"=w286, "RESULT_VALUE"=w276) -> ()  [unwired: 11 in, 1 out]
                  }
                }
              }
              frame #3 {
                n241 = global read "检测结果.vi" "合格状态"() -> (w295:string)
                n242 = local write "STEP"("自动" ("STEP")) -> ()
                n243 = case shown="\"合格\"" w295 {
                  frame "假", Default {
                  }
                  frame "合格" {
                    n244 = global read "Global.vi" "合格数量"() -> (w298:i32)
                    n245 = Increment(x=w298) -> (x+1=w297:i32)
                    n246 = global write "Global.vi" "合格数量"(w297) -> ()
                  }
                }
              }
            }
          }
        }
        n247 = global read "Global.vi" "程序关闭"() -> (w26:bool)
      }
      n248 = while {
        shift-right: [w299] -> w23
        shift-left: w24 -> [w300]
        stop <- w301 stop-if-true
        n249 = event shown="[7] \"0°曲线\", \"侧铆曲线\", \"45°曲线\", \"拉压曲线\", \"功能试验\", \"逆向空载试验\", \"磨合\": 鼠标按下" {
          selector: w300 -> [_ _ _ _ _ _ _ _]
          dyn-events: [_ _ _ _ _ _ _ _] -> w299
          timeout: 200 -> [_ _ _ _ _ _ _ _]
          event Timeout {
            n250 = event-data() -> ()  [unwired: 1 in, 3 out]
            n251 = call "Obtain Broadcast Events for Registration.vi"() -> ("Already running?"=w303:bool)  [unwired: 9 in, 2 out]
            n252 = case shown="真" w303 {
              frame False {
                n253 = local write "STEP"("手动" ("STEP")) -> ()
              }
              frame True {
                n254 = call "错误代码.vi"() -> ("Status_Read"=w305:u32)  [unwired: 11 in]
                n255 = feedback #1() -> (w315:u32)  [unwired: 1 in]
                n256 = feedback-in #1(w305) -> ()
                n257 = case shown="0" w305 {
                  frame 0 {
                    n258 = global read "Global.vi" "报警图标"() -> (w316:refnum<vi>)
                    n259 = property class="Bool"(reference=w316, "Visible"=FALSE ("可见")) -> ()  [unwired: 1 in, 2 out]
                  }
                  frame 1, Default {
                    n260 = global read "Global.vi" "报警图标"() -> (w319:refnum<vi>)
                    n261 = property class="Bool"(reference=w319, "Visible"=TRUE ("可见")) -> ()  [unwired: 1 in, 2 out]
                  }
                }
                n262 = Greater Or Equal?(x=w305, y=i16 5000) -> (x >= y?=w313:bool)
                n263 = Less?(x=w305, y=i16 5200) -> (x < y?=w314:bool)
                n264 = Equal?(x=w305, y=w315) -> (x = y?=w312:bool)
                n265 = global read "Global.vi" "报警图标"() -> (w307:refnum<vi>)
                n266 = And(x=w313, y=w314) -> (x .and. y?=w306:bool)
                n267 = property class="Bool"(reference=w307, "Value"=w306) -> ()  [unwired: 1 in, 2 out]
                n268 = Bundle By Name(cluster=errorcluster {"status"=FALSE, "code"=0, "source"=""} ("错误常量"), "status"=w306, "code"=w305) -> (w311:errorcluster)
                n269 = case shown="假" w312 {
                  tunnel: w311 -> [w320 _]
                  frame False {
                    n270 = call "报警处理.vi"("错误常量"=w320) -> ()  [unwired: 9 in, 2 out]
                  }
                  frame True {
                  }
                }
              }
            }
          }
          event User Event {
            n271 = event-data() -> ("试验项目"=w321:T1)  [unwired: 1 in]
            "试验项目" <- w321
            n272 = disable-structure shown="禁用" {
              disable-tunnel: w321 -> [w322 _]
              frame Disabled {
                n273 = global read "A180648.vi" "检测结果"() -> (w325:string[][][])
                n274 = global read "Global.vi" "Result"() -> (w323:refnum<vi>)
                n275 = Index Array(array=w325, index (dim 0)=w322) -> (element=w324:string[][])  [unwired: 2 in]
                n276 = property class="Tbl"(reference=w323, "Value"=w324) -> ()  [unwired: 1 in, 2 out]
              }
              frame Enabled {
              }
            }
          }
          event "试验项目": Value Change {
            n277 = event-data() -> ("NewVal"=w326:T1)  [unwired: 1 in]
            n278 = disable-structure shown="禁用" {
              disable-tunnel: w326 -> [w330 _]
              frame Disabled {
                n279 = global read "A180648.vi" "检测结果"() -> (w329:string[][][])
                n280 = global read "Global.vi" "Result"() -> (w327:refnum<vi>)
                n281 = Index Array(array=w329, index (dim 0)=w330) -> (element=w328:string[][])  [unwired: 2 in]
                n282 = property class="Tbl"(reference=w327, "Value"=w328) -> ()  [unwired: 1 in, 2 out]
              }
              frame Enabled {
              }
            }
          }
          event "0°曲线", "侧铆曲线", "45°曲线", "拉压曲线", "功能试验", "逆向空载试验", "磨合": Scale Range Change {
            n283 = event-data() -> ("CtlRef"=w332:refnum<vi>)  [unwired: 1 in, 4 out]
            n284 = global read "Global.vi" "产品型号"() -> (w331:string)
            n285 = call "XY_conf.vi"("方式"=enum16{"写入", "读取"}."写入", "产品"=w331, "XY图引用"=w332) -> ()  [unwired: 4 in, 1 out]
          }
          event User Event {
            n286 = event-data() -> ("产品"=w336:string)  [unwired: 1 in]
            n287 = control-ref of="0°曲线"() -> (w335:refnum<vi>)
            n288 = control-ref of="拉压曲线"() -> (w338:refnum<vi>)
            n289 = control-ref of="45°曲线"() -> (w334:refnum<vi>)
            n290 = control-ref of="侧铆曲线"() -> (w340:refnum<vi>)
            n291 = control-ref of="力特性试验"() -> (w339:refnum<vi>)
            n292 = Build Array(w335, w338, w334, w340, w339) -> (w337:refnum<vi>[])
            n293 = for {
              tunnel: w337 -> [w342] mode=indexing
              tunnel: w336 -> [w341]
              n294 = call "XY_conf.vi"("方式"=enum16{"写入", "读取"}."读取", "产品"=w341, "XY图引用"=w342) -> ()  [unwired: 4 in, 1 out]
            }
          }
          event Panel Close {
            n295 = event-data() -> ()  [unwired: 1 in, 4 out]
            n296 = global write "Global.vi" "程序关闭"(TRUE ("程序关闭")) -> ()
          }
          event "0°曲线", "侧铆曲线", "45°曲线", "拉压曲线", "功能试验", "逆向空载试验", "磨合": Mouse Enter; "0°曲线", "侧铆曲线", "45°曲线", "拉压曲线", "功能试验", "逆向空载试验", "磨合": Mouse Leave; "0°曲线", "侧铆曲线", "45°曲线", "拉压曲线", "功能试验", "逆向空载试验": Cursor Move; "磨合": Mouse Move {
            n297 = event-data() -> ("CtlRef"=w346:refnum<vi>, "Type"=w345:T8)  [unwired: 1 in]
            n298 = disable-structure shown="禁用" {
              disable-tunnel: w346 -> [w349 _]
              disable-tunnel: w345 -> [w347 _]
              frame Disabled {
                n299 = call "CursorShow.vi"("nameShow"=TRUE, "Type"=w347, "Graph"=w349) -> ()  [unwired: 7 in, 2 out]
              }
              frame Enabled {
              }
            }
          }
          event "0°曲线", "侧铆曲线", "45°曲线", "拉压曲线", "功能试验", "逆向空载试验", "磨合": Mouse Down {
            n300 = event-data() -> ("CtlRef"=w352:refnum<vi>, "Coords"=w351:T9, "Type"=w350:T8)  [unwired: 1 in]
            n301 = disable-structure shown="禁用" {
              disable-tunnel: w352 -> [w357 _]
              disable-tunnel: w351 -> [w356 _]
              disable-tunnel: w350 -> [w354 _]
              frame Disabled {
                n302 = invoke class="XYGraph (严格)" method="Map Coords To XY"(reference=w357, "Coords"=w356) -> (reference out=w355:refnum<vi>, "XY"=w353:cluster{"X":dbl, "Y":dbl})  [unwired: 5 in, 5 out]
                n303 = call "CursorShow.vi"("游标.游标位置"=w353, "Type"=w354, "Graph"=w355) -> ()  [unwired: 7 in, 2 out]
              }
              frame Enabled {
              }
            }
          }
        }
        n304 = global read "Global.vi" "程序关闭"() -> (w301:bool)
      }
    }
  }
  n305 = Unregister For Events(event registration refnum=w5) -> ()  [unwired: 1 in, 1 out]
